vi "UPS初始化变量(子VI).vi"(8 "error in (no error)":errorcluster) -> (0 "error out":errorcluster caption="错误输出")   [LabVIEW 2016, in "环境动力监测库.lvlib" / "UPS库.lvlib"]
uses:
  <vilib>/Utility/config.llb/NI_LVConfig.lvlib
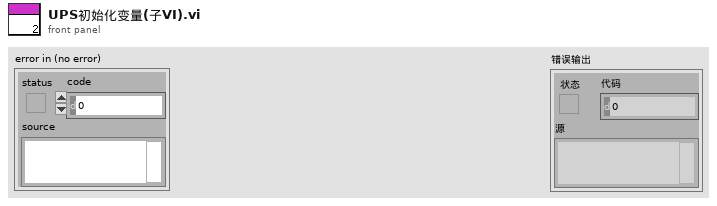
[diagram p1: front panel]
types:
  T1 = cluster{"监测项描述:输出":string, "连接方式":enum16{"串口", "TCP"}, "端口":string, "IP address:":string, "Port:":string, "站号":u64, "传感器型号":string, "波特率":u64, "data bits":u64, "停止位":u16, "奇偶校验":u16, "声光告警启用":bool}
  T2 = typedef "NI_LVConfig.lvlib/Config Data RefNum.ctl" = refnum<k1>
  T3 = typedef "环境动力监测库.lvlib/UPS库.lvlib/UPS型号.ctl" = enum16{"山特UPSC1~3", "山特UPSC6~20", "华为UPS2000-G-(1-3KVA)", "Kstar"}
  T4 = cluster{"VISA resource name":refnum<visa-resource-name>, "Serial Config":cluster{"baud rate (9600)":u32, "stop bits (10: 1 bit)":u16, "parity (0:none)":enum16{"None", "Odd", "Even", "Mark", "Space"}, "data bits (8)":u16, "timeout (10sec)":u32}, "型号选择":T3, "HW-UPS-2000 MB session":refnum<class "MB_Master.lvclass">, "连接方式":enum16{"串口", "TCP"}, "IP":string, "Port":string, "低电量报警阈值":u16, "功能启用":bool}
  T5 = cluster{"baud rate (9600)":u32, "stop bits (10: 1 bit)":u16, "parity (0:none)":enum16{"None", "Odd", "Even", "Mark", "Space"}, "data bits (8)":u16, "timeout (10sec)":u32}
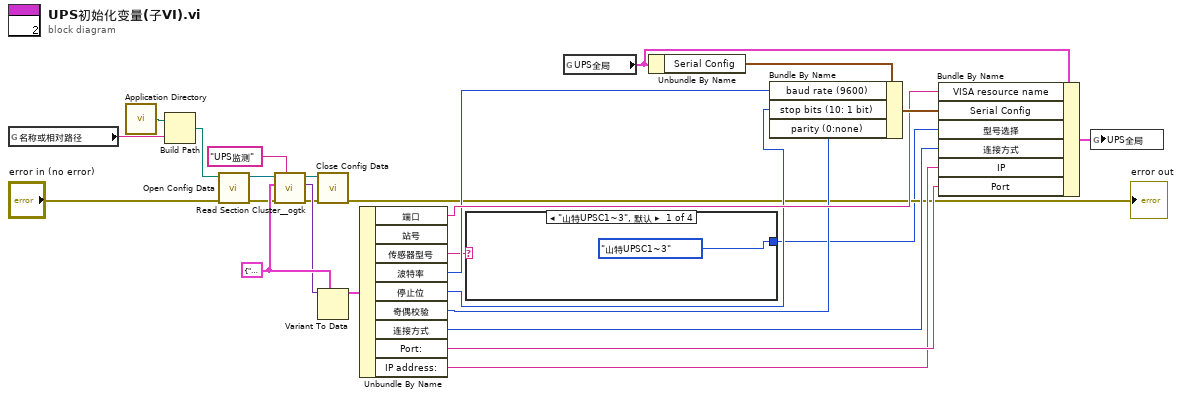
[diagram p0: block diagram]
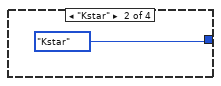
[diagram p2: hidden frame]
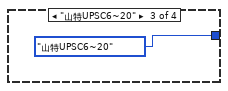
[diagram p3: hidden frame]
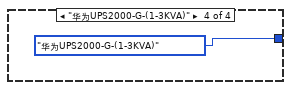
[diagram p4: hidden frame]
diagram:
  w13 = T1 {"监测项描述:输出"="", "连接方式"=enum."串口", "端口"="", "IP address:"="", "Port:"="", "站号"=19200, "传感器型号"="", "波特率"=19200, "data bits"=8, "停止位"=10, "奇偶校验"=0, "声光告警启用"=FALSE} ("输入簇")
  n1 = global read "内部交互全局变量.vi" "名称或相对路径"() -> (w2:string)
  n2 = call <vilib>:"Application Directory.vi"() -> ("Application Directory"=w8:path)
  n3 = Build Path(base path=w8, name or relative path=w2) -> (appended path=w7:path)
  n4 = call <vilib>:"Open Config Data.vi"("error in (no error)"="error in (no error)", "configuration file path"=w7) -> ("error out"=w6:errorcluster, "refnum"=w5:T2)  [unwired: 7 in, 1 out]
  n5 = call <userlib>:"Read Section Cluster__ogtk.vi"("section (optional)"="UPS监测", "error in (no error)"=w6, "Section Formatted Cluster Type"=w13, "refnum"=w5) -> ("error out"=w11:errorcluster, "Section Formatted Cluster"=w12:variant, "dup refnum"=w10:T2)  [unwired: 3 in, 2 out]
  n6 = call <vilib>:"Close Config Data.vi"("error in (no error)"=w11, "refnum"=w10) -> ("error out"=→"error out":errorcluster)  [unwired: 8 in, 1 out]
  n7 = Variant To Data(type=w13, Variant=w12) -> (data=w26:T1)  [unwired: 1 in, 1 out]
  n8 = Unbundle By Name(w26) -> ("端口"=w18:string, "传感器型号"=w14:string, "波特率"=w15:u64, "停止位"=w16:u16, "奇偶校验"=w17:u16, "连接方式"=w23:enum16{"串口", "TCP"}, "Port:"=w25:string, "IP address:"=w24:string)  [unwired: 1 out]
  n9 = case shown="\"山特UPSC1~3\", 默认" w14 {
    tunnel: [UPS型号."山特UPSC1~3" ("型号选择") UPS型号."Kstar" ("型号选择") UPS型号."山特UPSC6~20" ("型号选择") UPS型号."华为UPS2000-G-(1-3KVA)" ("型号选择")] -> w1
    frame "山特UPSC1~3", Default {
    }
    frame "Kstar" {
    }
    frame "山特UPSC6~20" {
    }
    frame "华为UPS2000-G-(1-3KVA)" {
    }
  }
  n10 = global read "断电保存全局变量.vi" "UPS全局"() -> (w20:T4)
  n11 = Unbundle By Name(w20) -> ("Serial Config"=w21:T5)
  n12 = Bundle By Name(cluster=w21, "baud rate (9600)"=w15, "stop bits (10: 1 bit)"=w16, "parity (0:none)"=w17) -> (w19:T5)
  n13 = Bundle By Name(cluster=w20, "VISA resource name"=w18, "Serial Config"=w19, "型号选择"=w1, "连接方式"=w23, "IP"=w24, "Port"=w25) -> (w22:T4)
  n14 = global write "断电保存全局变量.vi" "UPS全局"(w22) -> ()
